vi "Distance Drive.vi"(7 "PID gains":T1={"proportional gain (Kc)"=1.0, "integral time (Ti, min)"=0.01, "derivative time (Td, min)"=0.0} {"derivative time (Td, min)" format="%.3f"; "integral time (Ti, min)" format="%.3f"; "proportional gain (Kc)" format="%.3f"}, 8 "Distance Tolerance":dbl, 9 "Y Min Output":dbl, 10 "Y Max Output":dbl, 11 "Distance Target":dbl) -> (0 "Finished?":bool, 2 "Y Output":dbl)   [LabVIEW 2016]
uses:
  Common Code/Utilities/Change Detect Double.vi
  <vilib>/addons/control/pid/pid.llb/PID (DBL).vi
  <vilib>/addons/control/pid/NI_PID_pid.lvlib
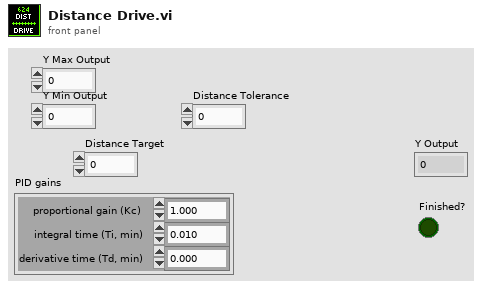
[diagram p1: front panel]
types:
  T1 = cluster{"proportional gain (Kc)":dbl, "integral time (Ti, min)":dbl, "derivative time (Td, min)":dbl}
  T2 = typedef "Drivetrain Encoder Values.ctl" = cluster{"Left Encoder":T3, "Center Encoder":T3, "Right Encoder":T3}
  T3 = typedef "Encoder Values.ctl" = cluster{"Distance":dbl, "Speed":dbl, "Tick":dbl}
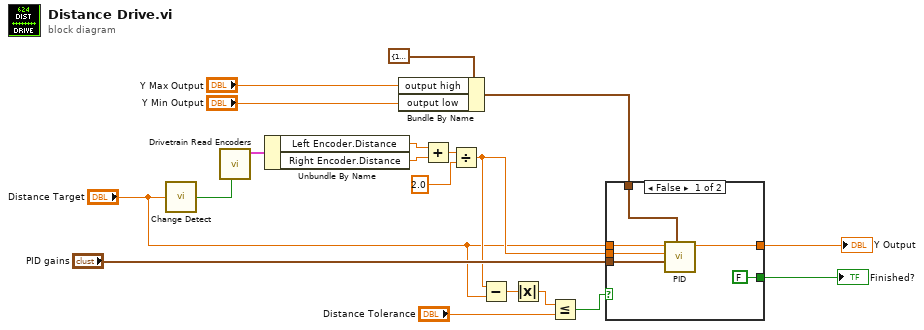
[diagram p0: block diagram]
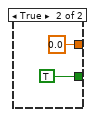
[diagram p2: hidden frame]
diagram:
  n1 = call-poly "Change Detect.vi"("In"="Distance Target") -> ("Changed?"=w19:bool)
  n2 = call "Drivetrain Read Encoders.vi"("Reset Encoders"=w19) -> ("Drivetrain Encoder Values"=w17:T2)  [unwired: 10 in]
  n3 = Unbundle By Name(w17) -> ("Left Encoder.Distance"=w16:dbl, "Right Encoder.Distance"=w15:dbl)
  n4 = Bundle By Name(cluster=cluster{"output high":dbl, "output low":dbl} {"output high"=100.0, "output low"=-100.0} ("output range"), "output high"="Y Max Output", "output low"="Y Min Output") -> (w10:cluster{"output high":dbl, "output low":dbl})
  n5 = Add(x=w16, y=w15) -> (x+y=w14:dbl)
  n6 = Divide(x=w14, y=2.0) -> (x/y=w8:dbl)
  n7 = Subtract(x=w8, y="Distance Target") -> (x-y=w6:dbl)
  n8 = Absolute Value(x=w6) -> (abs(x)=w5:dbl)
  n9 = Less Or Equal?(x=w5, y="Distance Tolerance") -> (x <= y?=w3:bool)
  n10 = case shown="False" w3 {
    tunnel: [w25 0.0 ("output")] -> w18
    tunnel: w8 -> [w24 _]
    tunnel: "Distance Target" -> [w23 _]
    tunnel: "PID gains" -> [w22 _]
    tunnel: w10 -> [w21 _]
    tunnel: [FALSE TRUE] -> w2
    frame False {
      n11 = call-poly <vilib>:"PID.vi"("output range"=w21, "PID gains"=w22, "process variable"=w24, "setpoint"=w23) -> ("output"=w25:dbl)  [unwired: 6 in, 1 out]
    }
    frame True {
    }
  }
  "Y Output" <- w18
  "Finished?" <- w2
